vi "Actuator Output Calculations.vi"(9 "Interval":dbl, 10 "CV1 Voltage":dbl, 11 "CV2 Voltage":dbl) -> (1 "Motor Speed":dbl, 2 "CV1 Flow Rate":dbl, 3 "CV2 Flow Rate":dbl)   [LabVIEW 2018]
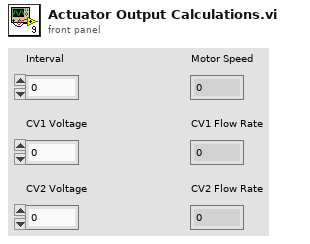
[diagram p1: front panel]
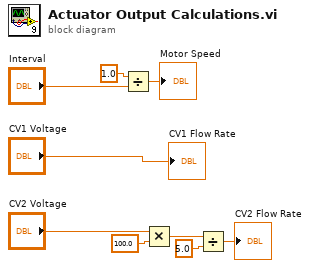
[diagram p0: block diagram]
diagram:
  n1 = Divide(x=1.0, y="Interval") -> (x/y=→"Motor Speed":dbl)
  n2 = Multiply(x="CV2 Voltage", y=100.0) -> (x*y=w2:dbl)
  n3 = Divide(x=w2, y=5.0) -> (x/y=→"CV2 Flow Rate":dbl)
  "CV1 Flow Rate" <- "CV1 Voltage"
